vi "Add New Events.vi"(6 "ms timeout (200)":i32=200, 7 "Event Names":string[](array[string]), 8 "queue":T1, 9 "Menu Refnum":refnum<k9>, 10 "New Events":bool[](array[boolean]), 11 "Event Queue In":string[](array[string])) -> (3 "Event Queue Out":string[](array[string]))   [LabVIEW 2017]
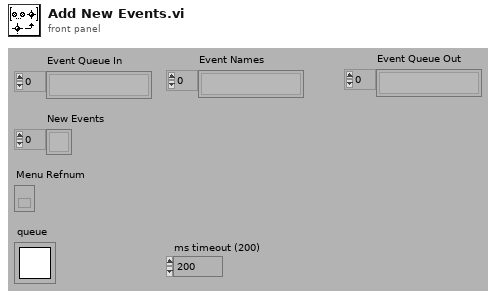
[diagram p1: front panel]
types:
  T1 = typedef "Queue RefNum" = refnum<k1>
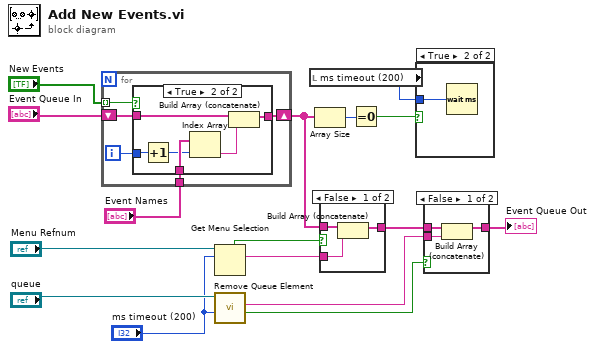
[diagram p0: block diagram]
diagram:
  n1 = for {
    shift-right: [w19] -> w4
    shift-left: "Event Queue In" -> [w20]
    tunnel: "New Events" -> [w18] mode=indexing
    tunnel: "Event Names" -> [w17]
    i -> [w21]
    n2 = case shown="True" w18 {
      tunnel: w21 -> [_ w24]
      tunnel: w20 -> [w22 w28]
      tunnel: [w22 w27] -> w19
      tunnel: w17 -> [_ w25]
      frame False {
      }
      frame True {
        n3 = Increment(x=w24) -> (x+1=w23:i32)
        n4 = Index Array(array=w25, index=w23) -> (element=w26:string)
        n5 = Build Array (concatenate)(w28, w26) -> (w27:string[])
      }
    }
  }
  n6 = Get Menu Selection(0:"Menu Refnum", 1:"ms timeout (200)") -> (4:w11:bool, 6:w9:string)  [unwired: 2 in, 3 out]
  n7 = call <vilib>:"Remove Queue Element.vi"("ms timeout (-1)"="ms timeout (200)", "queue"="queue") -> ("timed out"=w7:bool, "queue element"=w10:string)  [unwired: 4 in, 2 out]
  n8 = local read "ms timeout (200)"() -> (w1:i32)
  n9 = Array Size(array=w4) -> (size(s)=w3:i32)
  n10 = case shown="False" w11 {
    tunnel: w4 -> [w31 w32]
    tunnel: w9 -> [w30 _]
    tunnel: [w29 w32] -> w8
    frame False {
      n11 = Build Array (concatenate)(w31, w30) -> (w29:string[])
    }
    frame True {
    }
  }
  n12 = Equal To 0?(x=w3) -> (x = 0?=w2:bool)
  n13 = case shown="True" w2 {
    tunnel: w1 -> [_ w33]
    frame False {
    }
    frame True {
      n14 = Wait (ms)(milliseconds to wait=w33) -> ()  [unwired: 1 out]
    }
  }
  n15 = case shown="False" w7 {
    tunnel: w8 -> [w36 w37]
    tunnel: w10 -> [w35 _]
    tunnel: [w34 w37] -> w6
    frame False {
      n16 = Build Array (concatenate)(w36, w35) -> (w34:string[])
    }
    frame True {
    }
  }
  "Event Queue Out" <- w6
